vi "战斗.vi"() -> ()   [LabVIEW 2013]
panel:
  out "集气攻击":bool
  out "人神":i32(slide) scale=0.0..100.0
  out "人血条":i32(slide) scale=0.0..200.0
  out "还神丹":bool
  out "止血草":bool
  out "布尔":bool
  in  "枚举":enum16{"逃跑", "物品", "仙术", "攻击"}(ring)
  in  "逃跑1":cluster{"确定按钮":bool, "确定按钮 2":bool, "撤销":bool}
  in  "物品1":cluster{"确定按钮":bool, "确定按钮 2":bool, "撤销":bool}
  in  "攻击1":cluster{"普通攻击":bool, "集气攻击":bool, "撤销":bool}
  in  "仙术1":cluster{"确定按钮":bool, "确定按钮 2":bool, "撤销":bool}
  in  "逃跑":bool
  in  "物品":bool
  in  "仙术":bool
  in  "攻击":bool
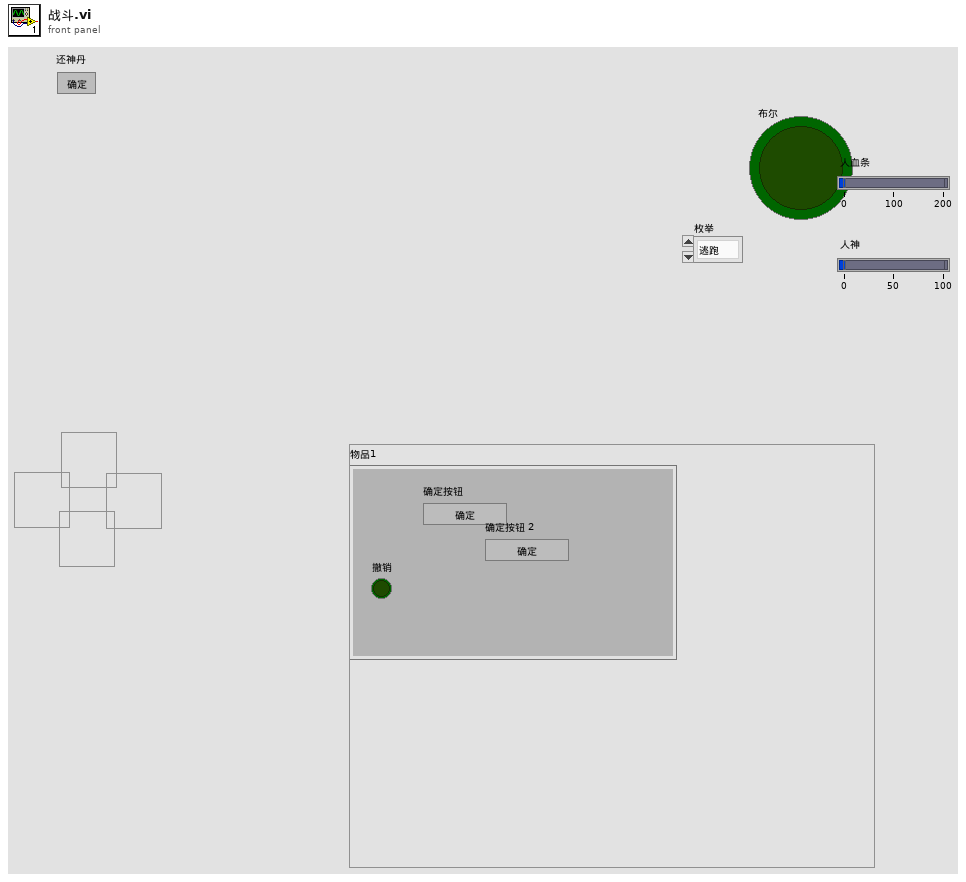
[diagram p1: front panel]
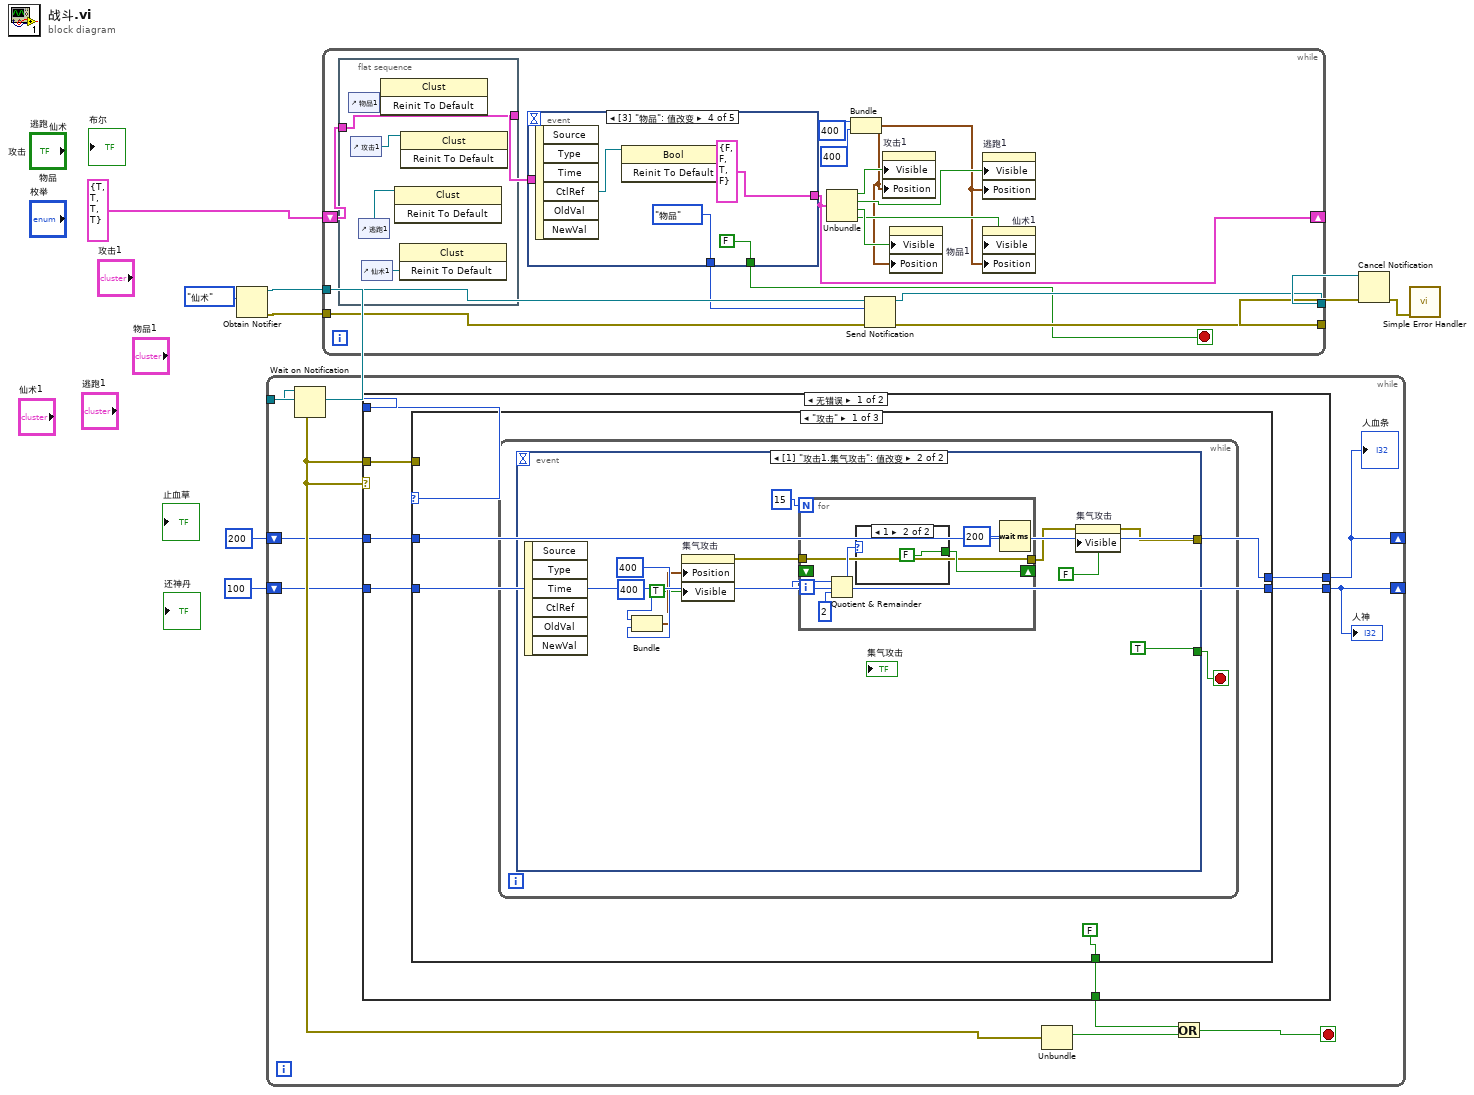
[diagram p0: block diagram]
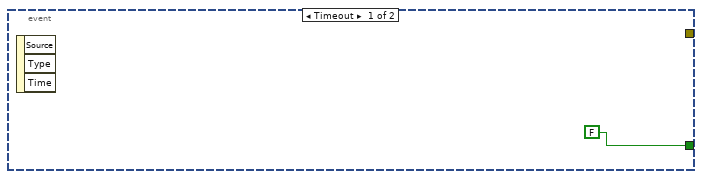
[diagram p2: hidden frame]
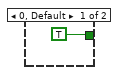
[diagram p3: hidden frame]
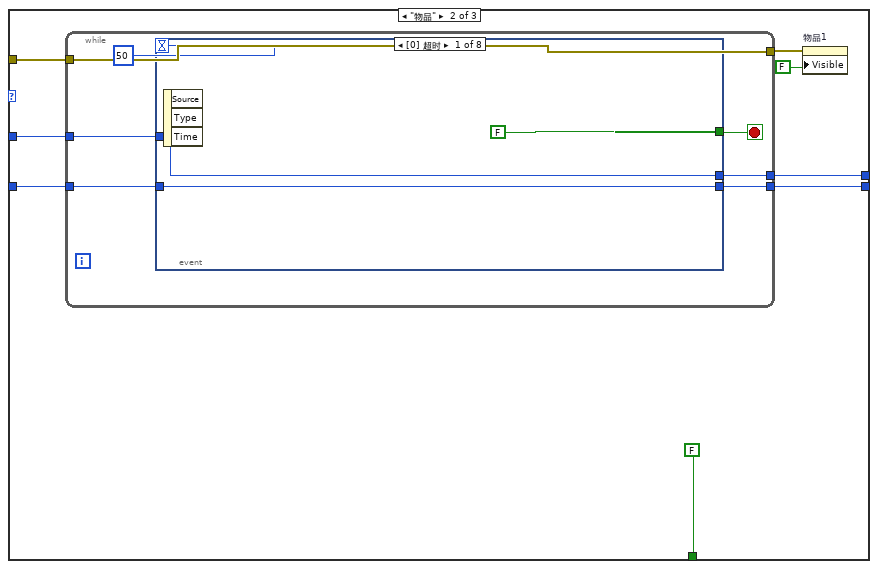
[diagram p4: hidden frame]
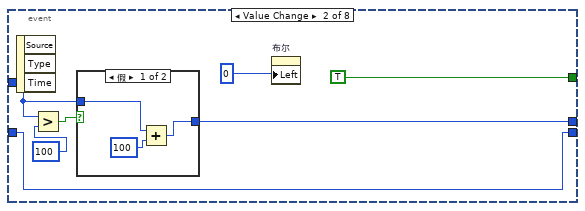
[diagram p5: hidden frame]
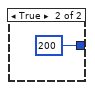
[diagram p6: hidden frame]
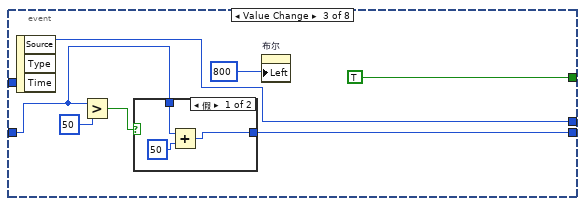
[diagram p7: hidden frame]
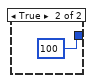
[diagram p8: hidden frame]
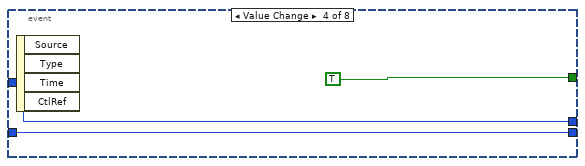
[diagram p9: hidden frame]
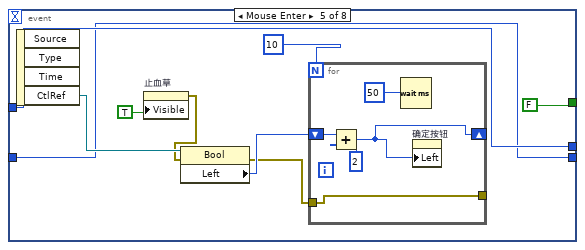
[diagram p10: hidden frame]
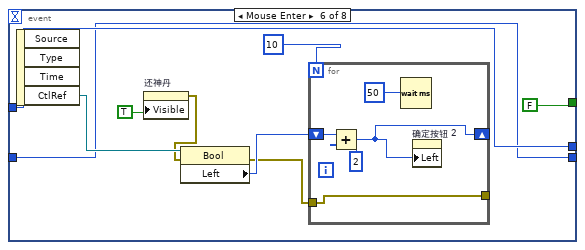
[diagram p11: hidden frame]
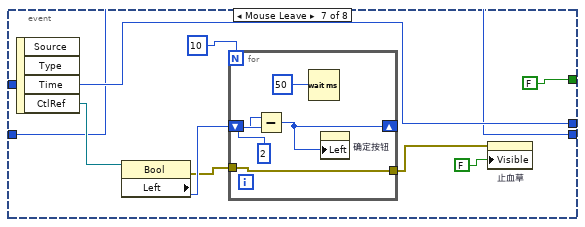
[diagram p12: hidden frame]
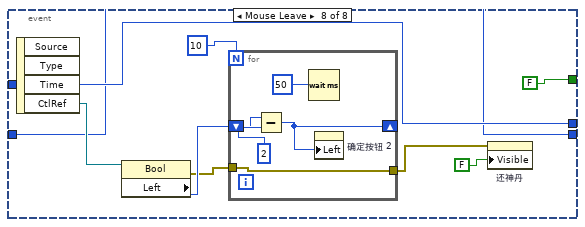
[diagram p13: hidden frame]
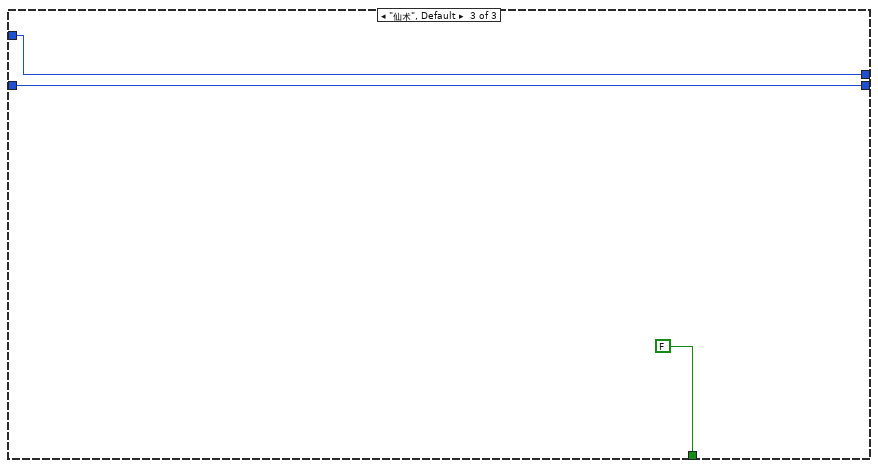
[diagram p14: hidden frame]
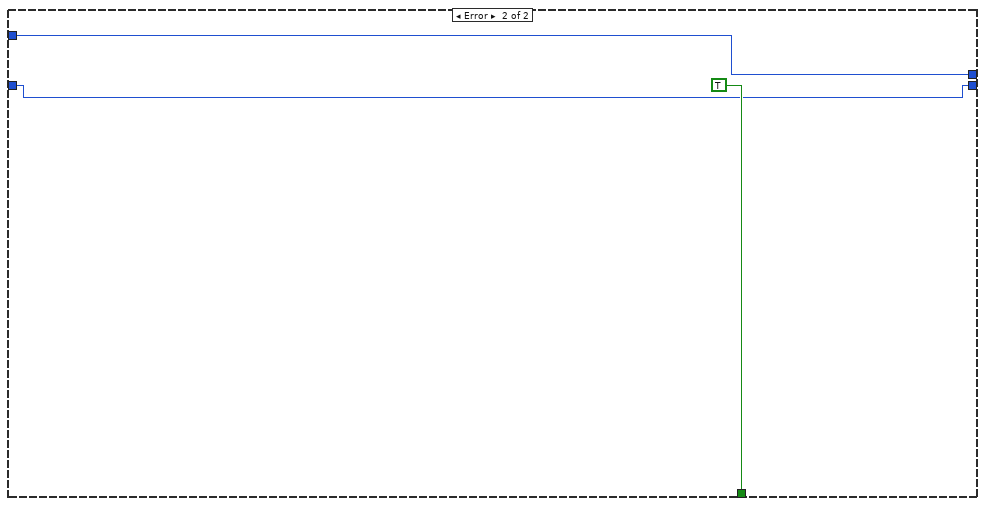
[diagram p15: hidden frame]
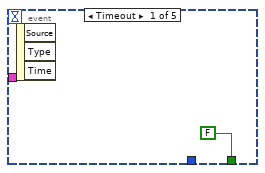
[diagram p16: hidden frame]
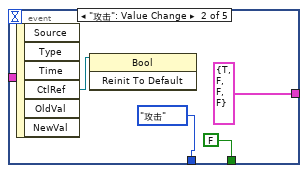
[diagram p17: hidden frame]
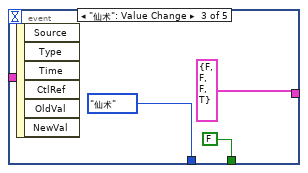
[diagram p18: hidden frame]
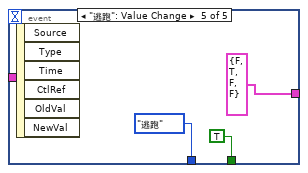
[diagram p19: hidden frame]
diagram:
  n1 = Obtain Notifier(notification data type=enum16{"逃跑", "物品", "仙术", "攻击"}."仙术" ("枚举")) -> (notifier out=w4:refnum<notifier>, error out=w9:errorcluster)  [unwired: 3 in, 1 out]
  n2 = while {
    tunnel: w4 -> [w19]
    shift-right: [w10] -> _
    shift-left: 200 -> [w13]
    shift-right: [w11] -> _
    shift-left: 100 -> [w12]
    stop <- w14 stop-if-true
    n3 = Wait on Notification(notifier=w19) -> (notification=w18:enum16{"逃跑", "物品", "仙术", "攻击"}, error out=w17:errorcluster)  [unwired: 3 in, 2 out]
    n4 = case shown="无错误" w17 {
      tunnel: w18 -> [w26 _]
      tunnel: w17 -> [w25 _]
      tunnel: [w24 TRUE] -> w16
      tunnel: w13 -> [w23 w153]
      tunnel: [w22 w153] -> w10
      tunnel: w12 -> [w21 w152]
      tunnel: [w20 w152] -> w11
      frame No Error {
        n5 = case shown="\"攻击\"" w26 {
          tunnel: w25 -> [_ w57 _]
          tunnel: [FALSE FALSE FALSE] -> w24
          tunnel: w23 -> [w28 w53 w151]
          tunnel: [w28 w52 w151] -> w22
          tunnel: w21 -> [w27 w51 w150]
          tunnel: [w27 w50 w150] -> w20
          frame "攻击" {
            n6 = while {
              stop <- w30 stop-if-true
              n7 = event shown="[1] \"攻击1.集气攻击\": 值改变" {
                selector: _ -> [_ _]
                dyn-events: _ -> [_ _]
                timeout: _ -> [_ _]
                tunnel: [FALSE TRUE] -> w30
                tunnel: [_ w32] -> _
                event Timeout {
                  n8 = event-data() -> ()  [unwired: 1 in, 3 out]
                }
                event "攻击1.集气攻击": Value Change {
                  n9 = event-data() -> ()  [unwired: 1 in, 6 out]
                  n10 = Bundle(400, 400) -> (w37:cluster{i32, i32})  [unwired: 1 in]
                  n11 = property on="集气攻击" class="Bool"("Position"=w37, "Visible"=TRUE ("可见")) -> (error out=w35:errorcluster)  [unwired: 2 in, 1 out]
                  n12 = for {
                    N: 15 -> [_]
                    shift-right: [w45] -> _
                    shift-left: _ -> [_]
                    tunnel: w35 -> [w42]
                    tunnel: [w42] -> w33
                    i -> [w43]
                    n13 = Quotient & Remainder(x=w43, y=2) -> (x-y*floor(x/y)=w46:i32)  [unwired: 1 out]
                    n14 = case shown="1" w46 {
                      tunnel: [TRUE FALSE] -> w45
                      frame 0, Default {
                      }
                      frame 1 {
                      }
                    }
                    n15 = Wait (ms)(milliseconds to wait=u32 200 ("等待时间（毫秒）")) -> ()  [unwired: 1 out]
                  }
                  n16 = property on="集气攻击" class="Bool"(error in=w33, "Visible"=FALSE) -> (error out=w32:errorcluster)  [unwired: 1 in, 1 out]
                }
              }
            }
          }
          frame "物品" {
            n17 = while {
              tunnel: w57 -> [w63]
              tunnel: [w63] -> w54
              tunnel: w53 -> [w61]
              tunnel: [w60] -> w52
              tunnel: w51 -> [w59]
              tunnel: [w58] -> w50
              stop <- w64 stop-if-true
              n18 = event shown="[0] 超时" {
                selector: _ -> [_ _ _ _ _ _ _ _]
                dyn-events: _ -> [_ _ _ _ _ _ _ _]
                timeout: 50 -> [_ _ _ _ _ _ _ _]
                tunnel: [FALSE TRUE TRUE TRUE FALSE FALSE FALSE FALSE] -> w64
                tunnel: w61 -> [w66 w69 w79 w91 w94 w108 w122 w136]
                tunnel: [w66 w70 w79 w91 w94 w108 w122 w136] -> w60
                tunnel: w59 -> [w65 w68 w81 w90 w93 w107 w121 w135]
                tunnel: [w65 w68 w80 w90 w93 w107 w121 w135] -> w58
                event Timeout {
                  n19 = event-data() -> ()  [unwired: 1 in, 3 out]
                }
                event "物品1.确定按钮": Value Change {
                  n20 = event-data() -> ()  [unwired: 1 in, 3 out]
                  n21 = Greater?(x=w69, y=100) -> (0:w71:bool)
                  n22 = case shown="假" w71 {
                    tunnel: [w75 200] -> w70
                    tunnel: w69 -> [w76 _]
                    frame False {
                      n23 = Add(x=w76, y=100) -> (x+y=w75:i32)
                    }
                    frame True {
                    }
                  }
                  n24 = property on="布尔" class="Bool (严格)"("Left"=0) -> ()  [unwired: 2 in, 2 out]
                }
                event "物品1.确定按钮 2": Value Change {
                  n25 = event-data() -> ()  [unwired: 1 in, 3 out]
                  n26 = Greater?(x=w81, y=50) -> (0:w82:bool)
                  n27 = case shown="假" w82 {
                    tunnel: [w86 100] -> w80
                    tunnel: w81 -> [w88 _]
                    frame False {
                      n28 = Add(x=w88, y=50) -> (x+y=w86:i32)
                    }
                    frame True {
                    }
                  }
                  n29 = property on="布尔" class="Bool (严格)"("Left"=800) -> ()  [unwired: 2 in, 2 out]
                }
                event "物品1.撤销": Value Change {
                  n30 = event-data() -> ()  [unwired: 1 in, 4 out]
                }
                event "物品1.确定按钮": Mouse Enter {
                  n31 = event-data() -> ("CtlRef"=w100:refnum<vi>)  [unwired: 1 in, 3 out]
                  n32 = property on="止血草" class="Bool (严格)"("Visible"=TRUE) -> (error out=w96:errorcluster)  [unwired: 2 in, 1 out]
                  n33 = property class="Bool"(reference=w100, error in=w96) -> (error out=w95:errorcluster, "Left"=w98:i32)  [unwired: 1 out]
                  n34 = for {
                    N: 10 -> [_]
                    shift-right: [w105] -> _
                    shift-left: w98 -> [w106]
                    tunnel: w95 -> [w102]
                    tunnel: [w102] -> _
                    n35 = Add(x=w106, y=2) -> (x+y=w105:i32)
                    n36 = Wait (ms)(milliseconds to wait=50) -> ()  [unwired: 1 out]
                    n37 = property on="确定按钮" class="Bool"("Left"=w105) -> ()  [unwired: 2 in, 2 out]
                  }
                }
                event "物品1.确定按钮 2": Mouse Enter {
                  n38 = event-data() -> ("CtlRef"=w114:refnum<vi>)  [unwired: 1 in, 3 out]
                  n39 = property on="还神丹" class="Bool (严格)"("Visible"=TRUE) -> (error out=w110:errorcluster)  [unwired: 2 in, 1 out]
                  n40 = property class="Bool"(reference=w114, error in=w110) -> (error out=w109:errorcluster, "Left"=w112:i32)  [unwired: 1 out]
                  n41 = for {
                    N: 10 -> [_]
                    shift-right: [w119] -> _
                    shift-left: w112 -> [w120]
                    tunnel: w109 -> [w116]
                    tunnel: [w116] -> _
                    n42 = Add(x=w120, y=2) -> (x+y=w119:i32)
                    n43 = Wait (ms)(milliseconds to wait=50) -> ()  [unwired: 1 out]
                    n44 = property on="确定按钮 2" class="Bool"("Left"=w119) -> ()  [unwired: 2 in, 2 out]
                  }
                }
                event "物品1.确定按钮": Mouse Leave {
                  n45 = event-data() -> ("CtlRef"=w127:refnum<vi>)  [unwired: 1 in, 3 out]
                  n46 = property class="Bool"(reference=w127) -> (error out=w124:errorcluster, "Left"=w128:i32)  [unwired: 1 in, 1 out]
                  n47 = for {
                    N: 10 -> [_]
                    shift-right: [w132] -> _
                    shift-left: w128 -> [w131]
                    tunnel: w124 -> [w130]
                    tunnel: [w130] -> w123
                    n48 = Subtract(x=w131, y=2) -> (x-y=w132:i32)
                    n49 = Wait (ms)(milliseconds to wait=50) -> ()  [unwired: 1 out]
                    n50 = property on="确定按钮" class="Bool"("Left"=w132) -> ()  [unwired: 2 in, 2 out]
                  }
                  n51 = property on="止血草" class="Bool (严格)"(error in=w123, "Visible"=FALSE) -> ()  [unwired: 1 in, 2 out]
                }
                event "物品1.确定按钮 2": Mouse Leave {
                  n52 = event-data() -> ("CtlRef"=w141:refnum<vi>)  [unwired: 1 in, 3 out]
                  n53 = property class="Bool"(reference=w141) -> (error out=w138:errorcluster, "Left"=w142:i32)  [unwired: 1 in, 1 out]
                  n54 = for {
                    N: 10 -> [_]
                    shift-right: [w146] -> _
                    shift-left: w142 -> [w145]
                    tunnel: w138 -> [w144]
                    tunnel: [w144] -> w137
                    n55 = Subtract(x=w145, y=2) -> (x-y=w146:i32)
                    n56 = Wait (ms)(milliseconds to wait=50) -> ()  [unwired: 1 out]
                    n57 = property on="确定按钮 2" class="Bool"("Left"=w146) -> ()  [unwired: 2 in, 2 out]
                  }
                  n58 = property on="还神丹" class="Bool (严格)"(error in=w137, "Visible"=FALSE) -> ()  [unwired: 1 in, 2 out]
                }
              }
            }
            n59 = property on="物品1" class="Clust"(error in=w54, "Visible"=FALSE) -> ()  [unwired: 1 in, 2 out]
          }
          frame "仙术", Default {
          }
        }
      }
      frame Error {
      }
    }
    "人血条" <- w10
    "人神" <- w11
    n60 = Unbundle(w17) -> ("status"=w15:bool)  [unwired: 2 out]
    n61 = Or(x=w16, y=w15) -> (x .or. y?=w14:bool)
  }
  n62 = while {
    tunnel: w4 -> [w170]
    tunnel: w9 -> [w169]
    shift-right: [w164] -> _
    shift-left: cluster{bool, bool, bool, bool} {TRUE, TRUE, TRUE, TRUE} -> [w156]
    tunnel: [w162] -> w6
    tunnel: [w161] -> w5
    stop <- w160 stop-if-true
    n63 = flat-sequence {
      tunnel: w156 -> [w174]
      tunnel: [w174] -> w155
      frame #0 {
        n64 = control-ref of="物品1"() -> (w175:refnum<vi>)
        n65 = control-ref of="攻击1"() -> (w173:refnum<vi>)
        n66 = control-ref of="逃跑1"() -> (w172:refnum<vi>)
        n67 = control-ref of="仙术1"() -> (w171:refnum<vi>)
        n68 = invoke class="Clust" method="Reinit To Default"(reference=w175) -> ()  [unwired: 2 in, 3 out]
        n69 = invoke class="Clust" method="Reinit To Default"(reference=w172) -> ()  [unwired: 2 in, 3 out]
        n70 = invoke class="Clust" method="Reinit To Default"(reference=w171) -> ()  [unwired: 2 in, 3 out]
        n71 = invoke class="Clust" method="Reinit To Default"(reference=w173) -> ()  [unwired: 2 in, 3 out]
      }
    }
    n72 = event shown="[3] \"物品\": 值改变" {
      selector: _ -> [_ _ _ _ _]
      dyn-events: _ -> [_ _ _ _ _]
      timeout: _ -> [_ _ _ _ _]
      tunnel: [_ cluster{bool, bool, bool, bool} {TRUE, FALSE, FALSE, FALSE} cluster{bool, bool, bool, bool} {FALSE, FALSE, FALSE, TRUE} cluster{bool, bool, bool, bool} {FALSE, FALSE, TRUE, FALSE} cluster{bool, bool, bool, bool} {FALSE, TRUE, FALSE, FALSE}] -> w164
      tunnel: [_ enum16{"逃跑", "物品", "仙术", "攻击"}."攻击" ("枚举") enum16{"逃跑", "物品", "仙术", "攻击"}."仙术" ("枚举") enum16{"逃跑", "物品", "仙术", "攻击"}."物品" ("枚举") enum16{"逃跑", "物品", "仙术", "攻击"}."逃跑" ("枚举")] -> w163
      tunnel: [FALSE FALSE FALSE FALSE TRUE] -> w160
      tunnel: w155 -> [_ _ _ _ _]
      event Timeout {
        n73 = event-data() -> ()  [unwired: 1 in, 3 out]
      }
      event "攻击": Value Change {
        n74 = event-data() -> ("CtlRef"=w177:refnum<vi>)  [unwired: 1 in, 5 out]
        n75 = invoke class="Bool" method="Reinit To Default"(reference=w177) -> ()  [unwired: 2 in, 3 out]
      }
      event "仙术": Value Change {
        n76 = event-data() -> ()  [unwired: 1 in, 6 out]
      }
      event "物品": Value Change {
        n77 = event-data() -> ("CtlRef"=w184:refnum<vi>)  [unwired: 1 in, 5 out]
        n78 = invoke class="Bool" method="Reinit To Default"(reference=w184) -> ()  [unwired: 2 in, 3 out]
      }
      event "逃跑": Value Change {
        n79 = event-data() -> ()  [unwired: 1 in, 6 out]
      }
    }
    n80 = Unbundle(w164) -> (w168:bool, w159:bool, w167:bool, w158:bool)
    n81 = Bundle(400, 400) -> (w157:cluster{i32, i32})  [unwired: 1 in]
    n82 = Send Notification(notification=w163, notifier=w170, error in (no error)=w169) -> (notifier out=w162:refnum<notifier>, error out=w161:errorcluster)
    n83 = property on="攻击1" class="Clust"("Visible"=w168, "Position"=w157) -> ()  [unwired: 2 in, 2 out]
    n84 = property on="物品1" class="Clust"("Visible"=w167, "Position"=w157) -> ()  [unwired: 2 in, 2 out]
    n85 = property on="逃跑1" class="Clust"("Visible"=w159, "Position"=w157) -> ()  [unwired: 2 in, 2 out]
    n86 = property on="仙术1" class="Clust"("Visible"=w158, "Position"=w157) -> ()  [unwired: 2 in, 2 out]
  }
  n87 = Cancel Notification(0:w6, 3:w5) -> (11:w3:errorcluster)  [unwired: 2 out]
  n88 = call <vilib>:"Simple Error Handler.vi"("error in (no error)"=w3) -> ()  [unwired: 4 in, 5 out]
